vi "Write E UI Refnum.vi"(8 "error in (no error)":errorcluster, 10 "E UI Refnum":refnum<vi>, 11 "HIJ JETI100 F and E Camera in":refnum<class "HIJ Vision App Fluence and Energy Camera.lvclass">) -> (0 "error out":errorcluster, 3 "HIJ JETI100 F and E Camera out":refnum<class "HIJ Vision App Fluence and Energy Camera.lvclass">)   [LabVIEW 2014, in "HIJ Vision App Fluence and Energy Camera.lvlib" / "HIJ Vision App Fluence and Energy Camera.lvclass"]
uses:
  HIJ Vision App Fluence and Energy Camera.lvclass
  HIJ Vision App Fluence and Energy Camera.lvclass/HIJ Vision App Fluence and Energy Camera.ctl
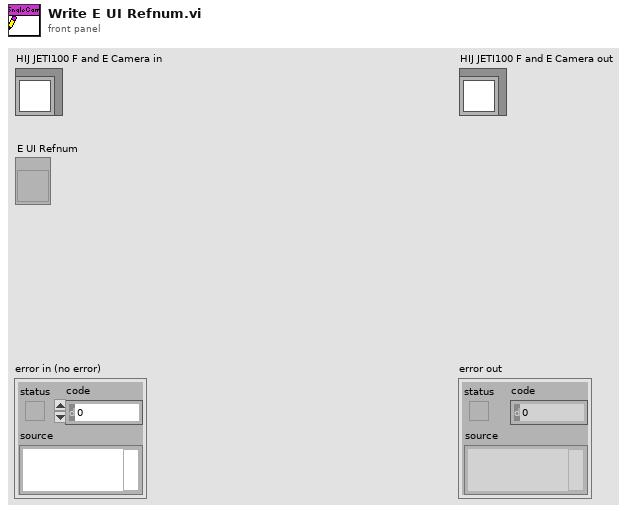
[diagram p1: front panel]
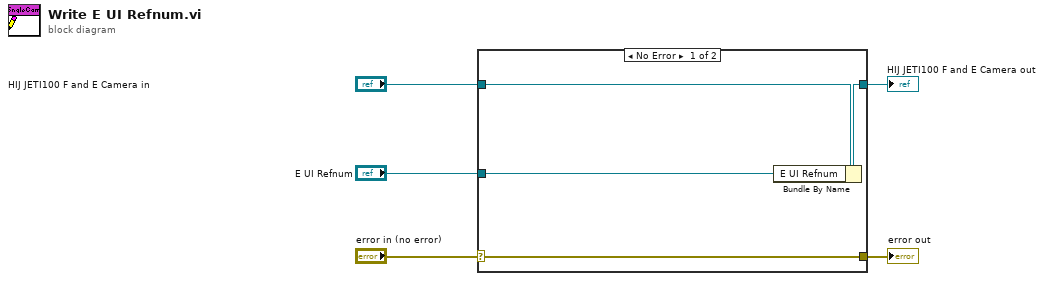
[diagram p0: block diagram]
diagram:
  n1 = case shown="No Error" "error in (no error)" {
    selector: "error in (no error)" -> [w9 w10]
    tunnel: [w9 w10] -> w4
    tunnel: [w7 w11] -> w2
    tunnel: "HIJ JETI100 F and E Camera in" -> [w8 w11]
    tunnel: "E UI Refnum" -> [w6 _]
    frame No Error {
      n2 = Bundle By Name(cluster=w8, "E UI Refnum"=w6) -> (w7:refnum<class "HIJ Vision App Fluence and Energy Camera.lvclass">)
    }
    frame Error {
    }
  }
  "error out" <- w4
  "HIJ JETI100 F and E Camera out" <- w2
